vi "MidBrainCommsTest.vi"() -> ()   [LabVIEW 2010]
uses:
  4-High Neurons/4.0-Super Heart Beat.ctl
  3-Midbrain/3.0-Global.vi
panel:
  in  "Stop Loops":bool
  out "4.7.4 - How UDP Server HB":T1
  out "4.7.4 How Server Error":errorcluster
  out "4.7.3 What Server Error":errorcluster
  out "4.7.3 - What UDP Server HB":T1
  out "4.7.2 Where Server Error":errorcluster
  out "4.7.2 - Where UDP Server HB":T1
  out "4.7.1 Act Client Error":errorcluster
  out "4.7.1 - Act UDP Client HB":T1
  in  "stop":bool
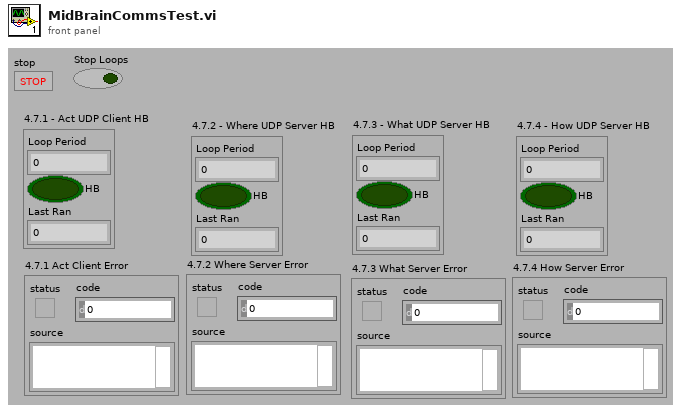
[diagram p1: front panel]
types:
  T1 = typedef "4.0-Super Heart Beat.ctl" = cluster{"Loop Period":u32, "HB":bool, "Last Ran":u32}
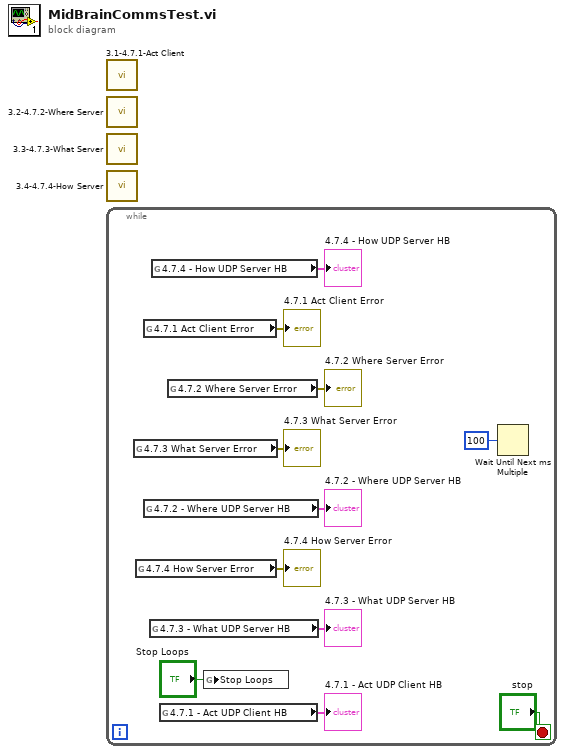
[diagram p0: block diagram]
diagram:
  n1 = call "3.1-4.7.1-Act Client.vi"() -> ()  [unwired: 12 in]
  n2 = call "3.2-4.7.2-Where Server.vi"() -> ()  [unwired: 12 in]
  n3 = call "3.3-4.7.3-What Server.vi"() -> ()  [unwired: 12 in]
  n4 = call "3.4-4.7.4-How Server.vi"() -> ()  [unwired: 1 in]
  n5 = while {
    stop <- "stop" stop-if-true
    n6 = global read "3.0-Global.vi" "4.7.3 What Server Error"() -> (→"4.7.3 What Server Error":errorcluster)
    n7 = global read "3.0-Global.vi" "4.7.4 How Server Error"() -> (→"4.7.4 How Server Error":errorcluster)
    n8 = global read "3.0-Global.vi" "4.7.1 Act Client Error"() -> (→"4.7.1 Act Client Error":errorcluster)
    n9 = global read "3.0-Global.vi" "4.7.2 - Where UDP Server HB"() -> (→"4.7.2 - Where UDP Server HB":T1)
    n10 = global read "3.0-Global.vi" "4.7.3 - What UDP Server HB"() -> (→"4.7.3 - What UDP Server HB":T1)
    n11 = global read "3.0-Global.vi" "4.7.4 - How UDP Server HB"() -> (→"4.7.4 - How UDP Server HB":T1)
    n12 = global read "3.0-Global.vi" "4.7.1 - Act UDP Client HB"() -> (→"4.7.1 - Act UDP Client HB":T1)
    n13 = global read "3.0-Global.vi" "4.7.2 Where Server Error"() -> (→"4.7.2 Where Server Error":errorcluster)
    n14 = global write "3.0-Global.vi" "Stop Loops"("Stop Loops") -> ()
    n15 = Wait Until Next ms Multiple(millisecond multiple=u32 100) -> ()  [unwired: 1 out]
  }
